vi "FGEN_Init.vi"(8 "Error In":errorcluster, 10 "HW Device Name":string, 11 "Object in":refnum<class "FGEN.lvclass">) -> (0 "Error Out":errorcluster, 3 "object out":refnum<class "FGEN.lvclass">)   [LabVIEW 2023, in "HAL.lvlib" / "FGEN.lvlib" / "FGEN.lvclass"]
uses:
  FGEN.lvclass
  D:/git/HAL/Hardware_class/Hardware.lvclass
  FGEN.lvclass/FGEN.ctl
  Hardware_class/Hardware.lvclass
  D:/git/HAL/FGEN_class/FGEN.lvclass
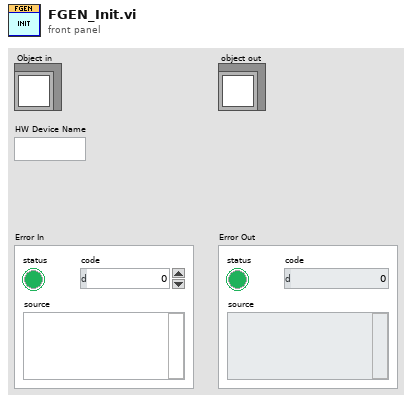
[diagram p1: front panel]
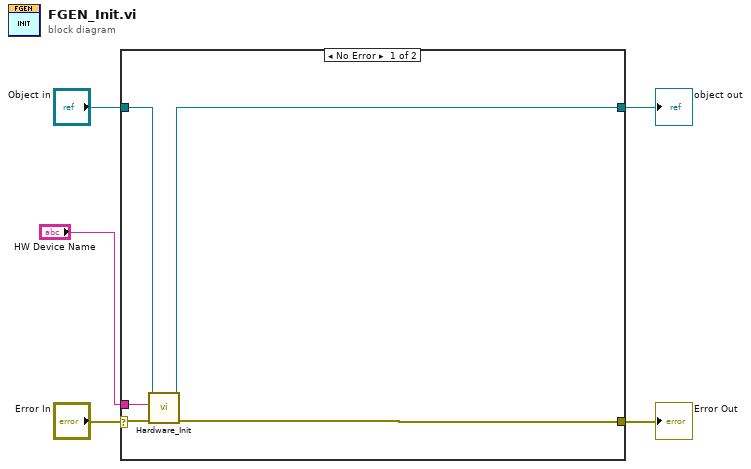
[diagram p0: block diagram]
diagram:
  n1 = case shown="No Error" "Error In" {
    selector: "Error In" -> [w10 w11]
    tunnel: [w6 w12] -> w5
    tunnel: "Object in" -> [w8 w12]
    tunnel: [w9 w11] -> w2
    tunnel: "HW Device Name" -> [w7 _]
    frame No Error {
      n2 = call "Hardware_Init.vi"("Error In"=w10, "HW Device Name"=w7, "object in"=w8) -> ("Error Out"=w9:errorcluster, "object out"=w6:refnum<class "FGEN.lvclass">)  [unwired: 7 in]
    }
    frame Error {
    }
  }
  "object out" <- w5
  "Error Out" <- w2
